vi "Hardware in the Loop - Configure Settings.vi"(10 "Samples to Read":i32=100000, 11 "Address":string) -> (0 "error out":errorcluster)   [LabVIEW 2017, in "Communications Library.lvlib"]
doc: "Configures the DTACQ device for hardware in the loop mode. \n\nSets the transient capture mode and trigger mode."
uses:
  Communications Library.lvlib
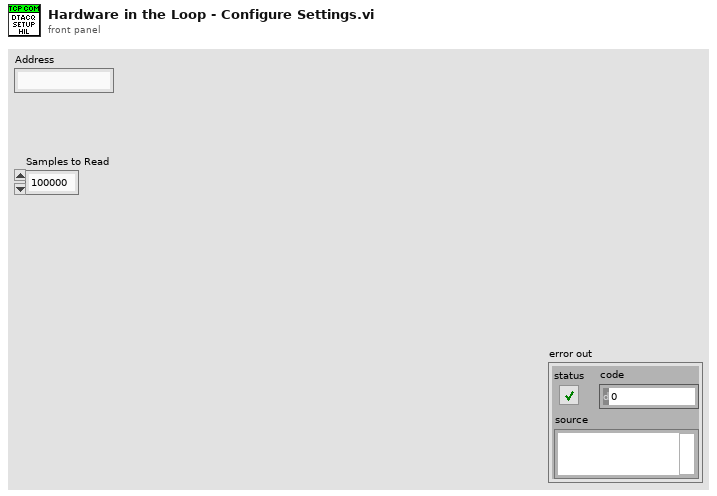
[diagram p1: front panel]
types:
  T1 = typedef "Communications Library.lvlib/DTACQ Connection Data--Cluster.ctl" = cluster{"Description":string, "Address":string, "Port":u16, "timeout (ms)":i32, "Termination Character":string, "TCP Connection Reference":refnum<k5>, "Open Connection":bool}
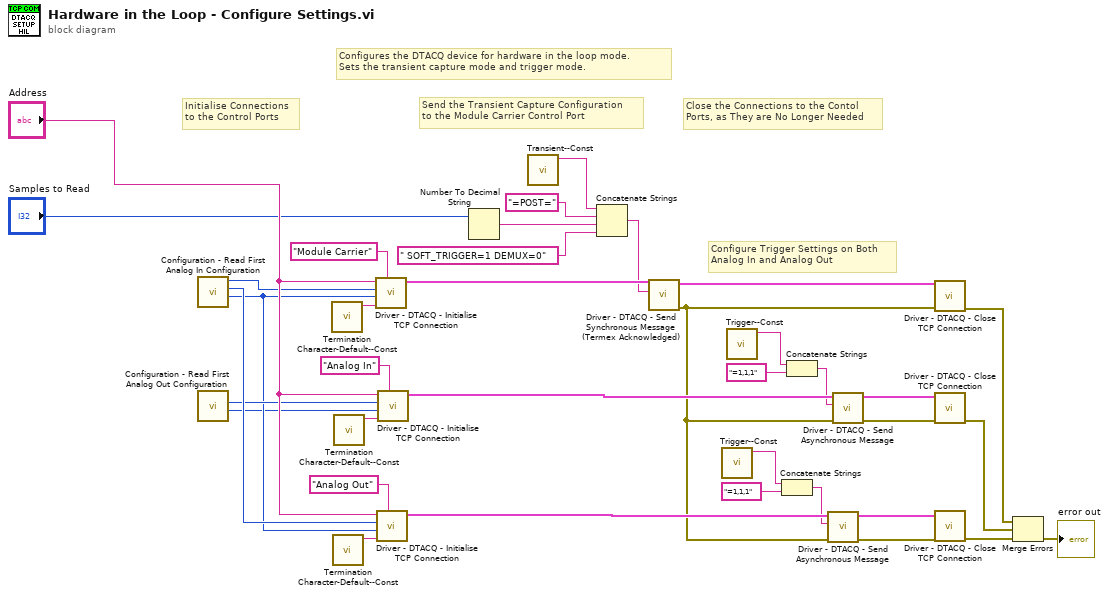
[diagram p0: block diagram]
diagram:
  # "Configures the DTACQ device for hardware in the loop mode.  \nSets the transient capture mode and trigger mode."
  # "Close the Connections to the Contol\nPorts, as They are No Longer Needed"
  # "Configure Trigger Settings on Both\nAnalog In and Analog Out"
  # "Send the Transient Capture Configuration\nto the Module Carrier Control Port"
  # "Initialise Connections\nto the Control Ports"
  n1 = call "Configuration - Read First Analog In Configuration.vi"() -> ("Timeout (ms)"=w2:i32, "Analog In Control Port"=w4:i32, "Carrier Control Port"=w5:i32)  [unwired: 7 in, 2 out]
  n2 = call "Configuration - Read First Analog Out Configuration.vi"() -> ("Timeout (ms)"=w1:i32, "Analog Out Control Port"=w3:i32)  [unwired: 7 in, 3 out]
  n3 = call "Termination Character-Default--Const.vi"() -> ("Termination Character"=w27:string)  [unwired: 11 in]
  n4 = call "Termination Character-Default--Const.vi"() -> ("Termination Character"=w23:string)  [unwired: 11 in]
  n5 = call "Termination Character-Default--Const.vi"() -> ("Termination Character"=w25:string)  [unwired: 11 in]
  n6 = call "Driver - DTACQ - Initialise TCP Connection.vi"("Description"="Module Carrier", "Termination Character"=w27, "timeout (ms)"=w2, "Port"=w5, "Address"="Address") -> ("DTACQ Connection Data Out"=w9:T1)  [unwired: 6 in]
  n7 = call "Driver - DTACQ - Initialise TCP Connection.vi"("Description"="Analog Out", "Termination Character"=w23, "timeout (ms)"=w2, "Port"=w4, "Address"="Address") -> ("DTACQ Connection Data Out"=w35:T1)  [unwired: 6 in]
  n8 = call "Driver - DTACQ - Initialise TCP Connection.vi"("Description"="Analog In", "Termination Character"=w25, "timeout (ms)"=w1, "Port"=w3, "Address"="Address") -> ("DTACQ Connection Data Out"=w36:T1)  [unwired: 6 in]
  n9 = Number To Decimal String(number="Samples to Read") -> (decimal integer string=w22:string)  [unwired: 1 in]
  n10 = call "Transient--Const.vi"() -> ("Transient Command"=w21:string)  [unwired: 11 in]
  n11 = Concatenate Strings(w21, "=POST=" ("string"), w22, " SOFT_TRIGGER=1 DEMUX=0" ("string")) -> (w8:string)
  n12 = call "Driver - DTACQ - Send Synchronous Message (Termex Acknowledged).vi"("Message to Send"=w8, "DTACQ Connection Data In"=w9) -> ("error out"=w6:errorcluster, "DTACQ Connection Data Out"=w7:T1)  [unwired: 6 in, 2 out]
  n13 = call "Trigger--Const.vi"() -> ("Trigger Command"=w13:string)  [unwired: 11 in]
  n14 = call "Trigger--Const.vi"() -> ("Trigger Command"=w18:string)  [unwired: 11 in]
  n15 = Concatenate Strings(w13, "=1,1,1" ("string")) -> (w14:string)
  n16 = Concatenate Strings(w18, "=1,1,1" ("string")) -> (w16:string)
  n17 = call "Driver - DTACQ - Send Asynchronous Message.vi"("error in"=w6, "Message to Send"=w14, "DTACQ Connection Data In"=w35) -> ("error out"=w30:errorcluster, "DTACQ Connection Data Out"=w31:T1)  [unwired: 7 in]
  n18 = call "Driver - DTACQ - Send Asynchronous Message.vi"("error in"=w6, "Message to Send"=w16, "DTACQ Connection Data In"=w36) -> ("error out"=w33:errorcluster, "DTACQ Connection Data Out"=w32:T1)  [unwired: 7 in]
  n19 = call "Driver - DTACQ - Close TCP Connection.vi"("error in"=w6, "DTACQ Connection Data In"=w7) -> ("error out"=w10:errorcluster)  [unwired: 8 in, 1 out]
  n20 = call "Driver - DTACQ - Close TCP Connection.vi"("error in"=w33, "DTACQ Connection Data In"=w32) -> ("error out"=w11:errorcluster)  [unwired: 8 in, 1 out]
  n21 = call "Driver - DTACQ - Close TCP Connection.vi"("error in"=w30, "DTACQ Connection Data In"=w31) -> ("error out"=w12:errorcluster)  [unwired: 8 in, 1 out]
  n22 = Merge Errors(w10, w11, w12) -> (→"error out":errorcluster)
